vi "Write Boder Spacing.vi"(3 "(FPSZ)":refnum<class "FPSZ.lvclass">, 4 "Border Spacing":i16) -> (5 "(FPSZ) Out":refnum<class "FPSZ.lvclass">)   [LabVIEW 2025, in "FPSZ.lvclass"]
uses:
  FPSZ.lvclass
  FPSZ.lvclass/FPSZ.ctl
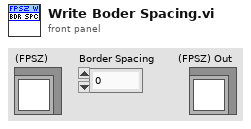
[diagram p1: front panel]
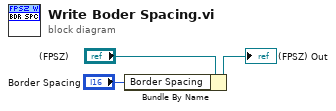
[diagram p0: block diagram]
diagram:
  n1 = Bundle By Name(cluster="(FPSZ)", "Border Spacing"="Border Spacing") -> (→"(FPSZ) Out":refnum<class "FPSZ.lvclass">)
